vi "Status Get Pressure and Flow Rate.vi"(5 "Retry Attempts (0)":i32 min=0, 7 "Fast Comms (F)":bool, 8 "error in":errorcluster, 11 "VISA resource name":refnum<visa-resource-name>) -> (0 "error out":errorcluster, 1 "Flow Rate":dbl, 2 "Pressure":dbl, 3 "VISA resource name out":refnum<visa-resource-name>)   [LabVIEW 2020, in "chromtech_nextgen_pump_drivers.lvlib"]
doc: "Queries the pump for current conditions of pressure and flow rate."
uses:
  chromtech_nextgen_pump_drivers.lvlib
panel:
  out "Response":string
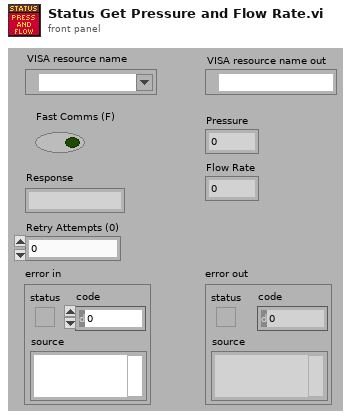
[diagram p1: front panel]
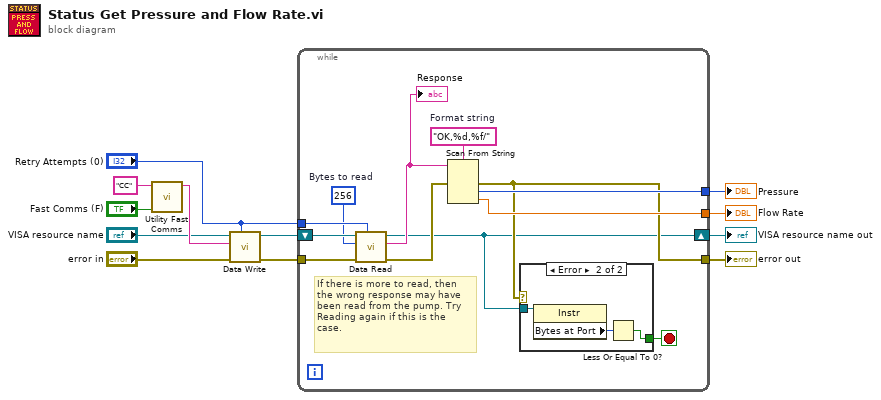
[diagram p0: block diagram]
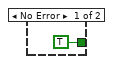
[diagram p2: hidden frame]
diagram:
  n1 = call "Utility Fast Comms.vi"("Fast Comms"="Fast Comms (F)", "Command"="CC") -> ("Fast Command"=w5:string)  [unwired: 9 in]
  n2 = call "Data Write.vi"("Retry Attempts (0)"="Retry Attempts (0)", "error in (no error)"="error in", "Command"=w5, "VISA Refnum in"="VISA resource name") -> ("error out"=w1:errorcluster, "VISA Refnum out"=w2:refnum<visa-resource-name>)  [unwired: 6 in]
  n3 = while {
    tunnel: [w24] -> w10
    tunnel: [w23] -> w9
    tunnel: "Retry Attempts (0)" -> [w22]
    shift-right: [w14] -> w7
    shift-left: w2 -> [w21]
    tunnel: w1 -> [w20]
    tunnel: [w15] -> w8
    stop <- w13 stop-if-true
    w18 = "OK,%d,%f/"  # Format string
    w19 = u32 256  # Bytes to read
    # "If there is more to read, then\nthe wrong response may have\nbeen read from the pump. Try\nReading again if this is the\ncase."
    n4 = call "Data Read.vi"("Retry Attempts (0)"=w22, "error in (no error)"=w20, "Bytes to read"=w19, "VISA Refnum in"=w21) -> ("error out"=w17:errorcluster, "read buffer"=w16:string, "VISA Refnum out"=w14:refnum<visa-resource-name>)  [unwired: 5 in]
    "Response" <- w16
    n5 = Scan From String(format string=w18, input string=w16, error in=w17) -> (error out=w15:errorcluster, output 1=w24:i32, output 2=w23:dbl)  [unwired: 3 in, 2 out]
    n6 = case shown="Error" w15 {
      tunnel: w14 -> [_ w28]
      tunnel: [TRUE w26] -> w13
      frame No Error {
      }
      frame Error {
        n7 = property class="Instr"(reference=w28) -> ("Bytes at Port"=w27:u32)  [unwired: 1 in, 2 out]
        n8 = Less Or Equal To 0?(x=w27) -> (x <= 0?=w26:bool)
      }
    }
  }
  "VISA resource name out" <- w7
  "error out" <- w8
  "Pressure" <- w10
  "Flow Rate" <- w9
